vi "Path Edit.vi"() -> ()   [LabVIEW 2016]
uses:
  typedefs/Schedule - enum.ctl
  Global Variables.vi
panel:
  in  "Index":i32=8
  in  "Direction":u16(ring) items=["Forward", "Backward"]
  in  "Enabled":bool=TRUE
  in  "Voltage Schedule":T1
  in  "Apply to All":bool
  in  "Fill Orientation":u16(ring) items=["Horizontal", "Vertical"]
  in  "Smooth Segments":dbl=12.0
  in  "Speed Schedule":T1
  in  "Speed (µm/s)":dbl=8.0
  in  "Voltage (V)":dbl=8.0
  in  "Speed Settings":bool
  in  "Voltage Settings":bool
  in  "Fill Spacing":dbl=0.1
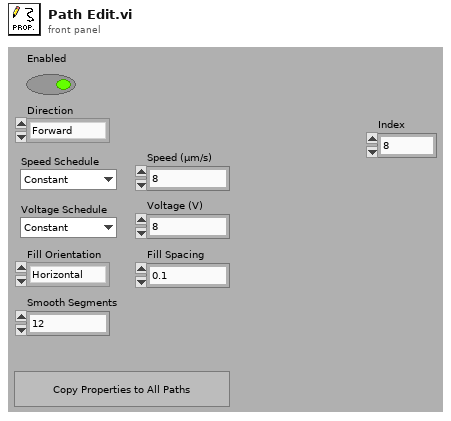
[diagram p1: front panel]
types:
  T1 = typedef "Schedule - enum.ctl" = enum16{"Constant", "Ramp", "Fn. Generator", "Formula"}
  T2 = enum32{"invalid app kind", "Development System", "Run Time System", "Student Edition", "Embedded LabVIEW", "Evaluation", "Custom"}
  T3 = enum32{"Invalid", "Standard", "Closed", "Hidden", "Minimized", "Maximized"}
  T4 = typedef "Path Properties - cluster.ctl" = cluster{"Enabled":bool, "Direction":u16, "Fill Orientation":u16, "Smooth Segments":dbl, "Fill Spacing":dbl, "Speed (um/s)":T5, "Voltage (V)":T5}
  T5 = typedef "Voltage - cluster.ctl" = cluster{"Schedule":T1, "Value":dbl, "Start Value":dbl, "End Value":dbl, "Min Value":dbl, "Max Value":dbl, "Duty Cycle (%)":dbl, "Signal Type":T6, "Cycle Number":dbl, "Phase (degrees)":dbl, "formula":string, "formula length (nm)":dbl, "formula resolution (nm)":dbl}
  T6 = typedef "Signal Type - enum.ctl" = enum16{"Sine Wave", "Triangle Wave", "Square Wave", "Sawtooth Wave"}
  T7 = cluster{"Core":cluster{"Current VI Reference":refnum<vi>, "Close Panel on Exit?":bool}}
  T8 = cluster{"Current VI Reference":refnum<vi>, "Close Panel on Exit?":bool}
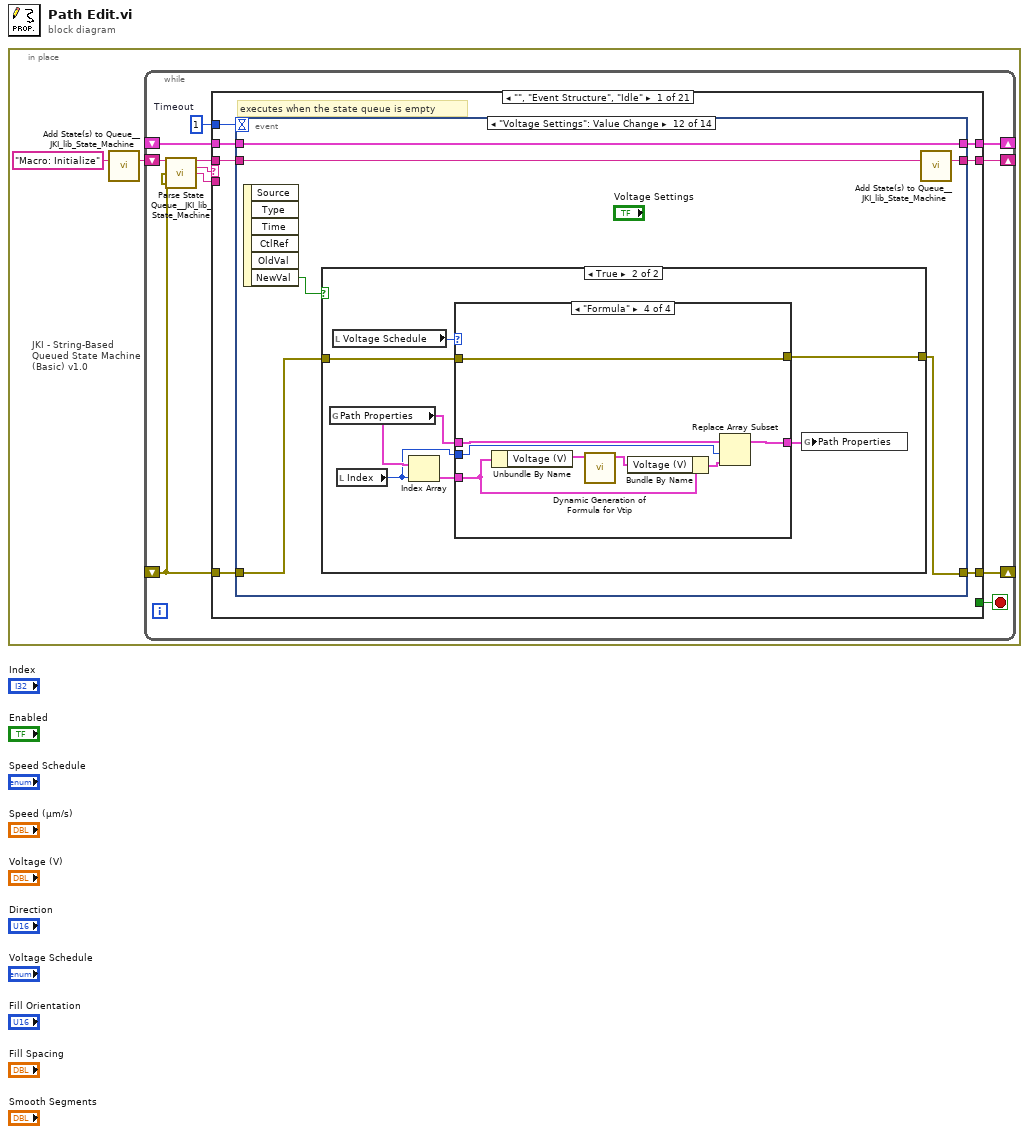
[diagram p0: block diagram]
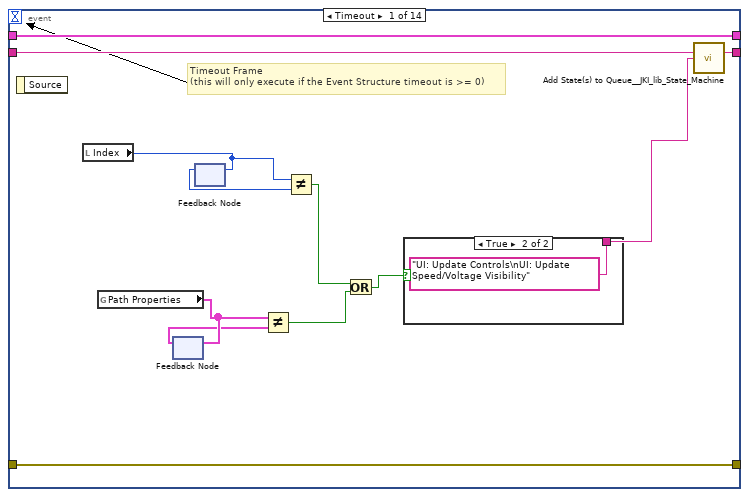
[diagram p2: hidden frame]
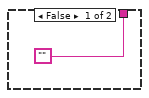
[diagram p3: hidden frame]
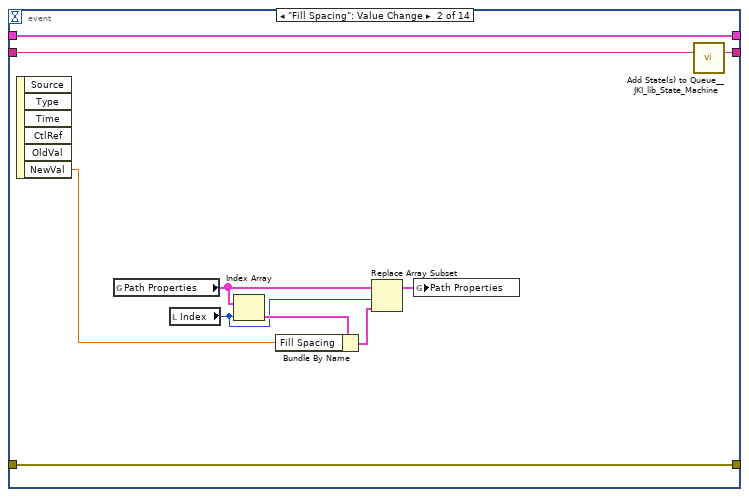
[diagram p4: hidden frame]
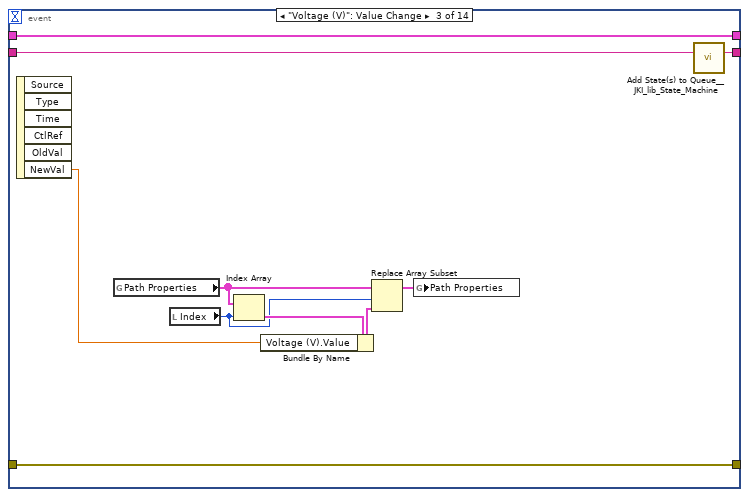
[diagram p5: hidden frame]
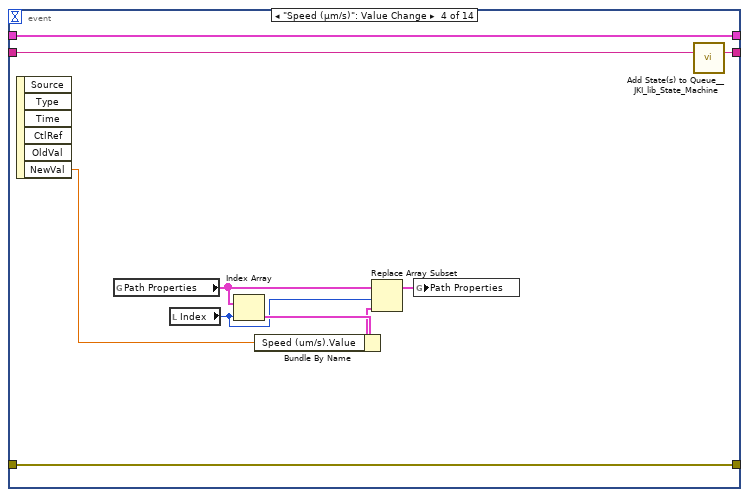
[diagram p6: hidden frame]
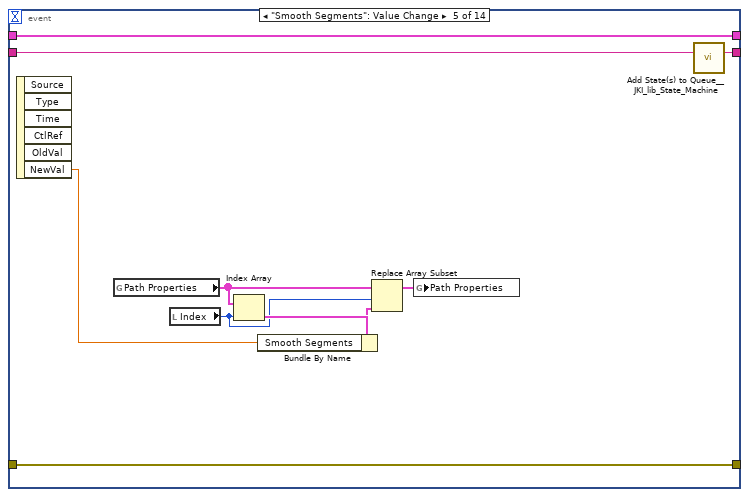
[diagram p7: hidden frame]
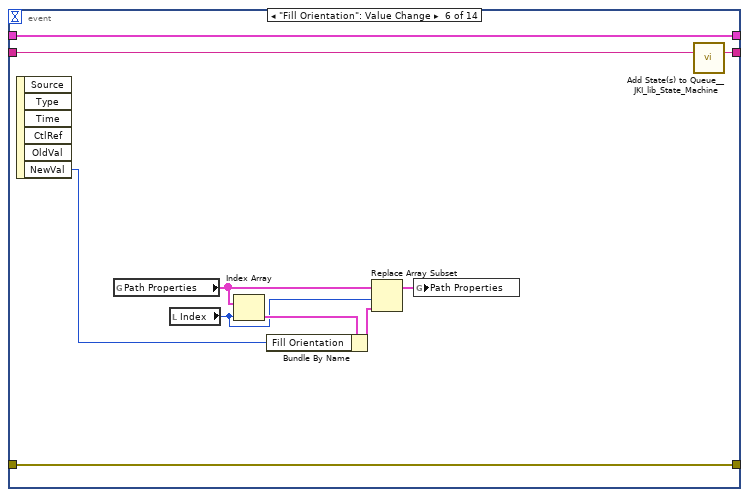
[diagram p8: hidden frame]
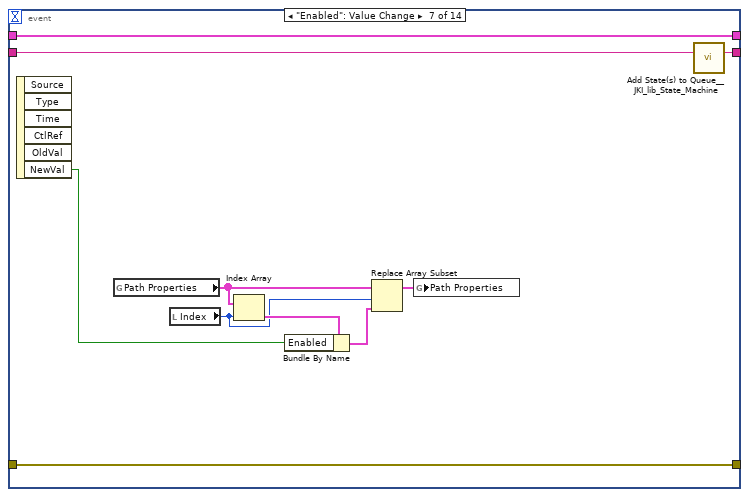
[diagram p9: hidden frame]
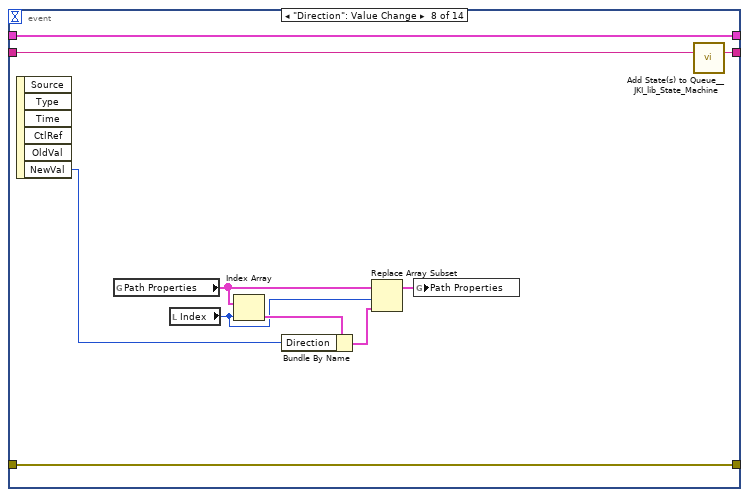
[diagram p10: hidden frame]
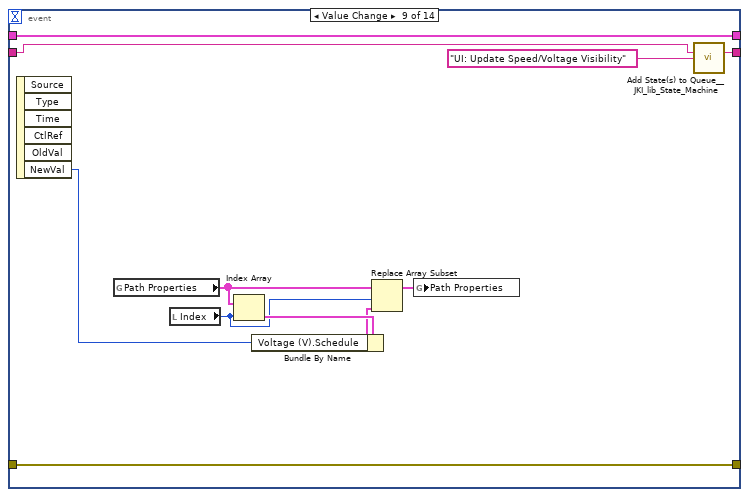
[diagram p11: hidden frame]
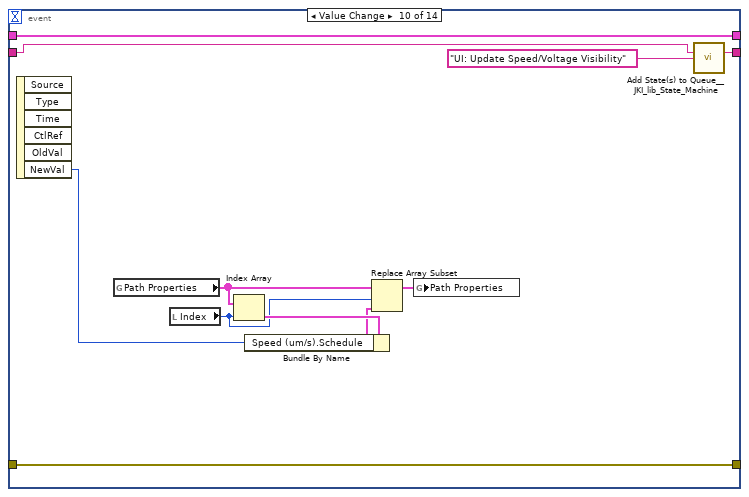
[diagram p12: hidden frame]
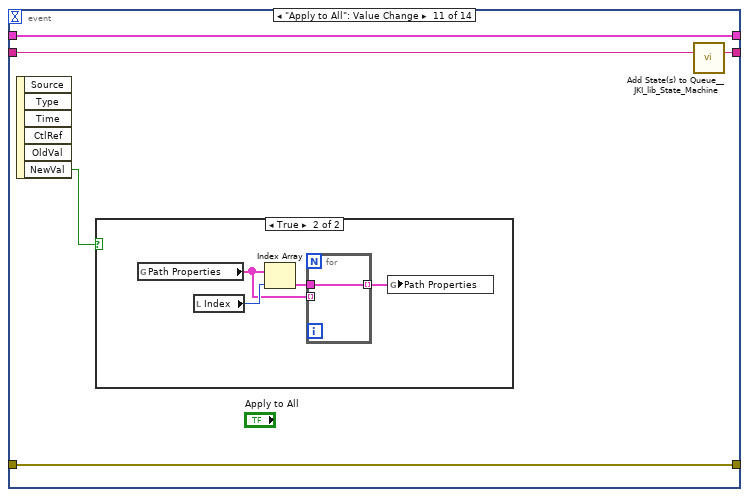
[diagram p13: hidden frame]
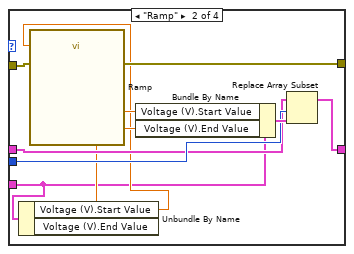
[diagram p17: hidden frame]
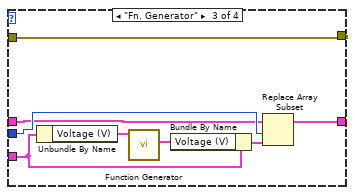
[diagram p18: hidden frame]
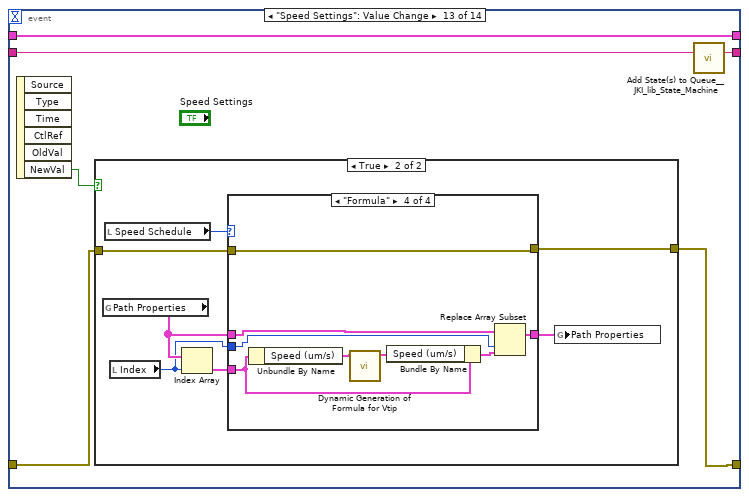
[diagram p19: hidden frame]
diagram:
  n1 = in-place {
    n2 = call <vilib>:"Add State(s) to Queue__JKI_lib_State_Machine.vi"("State(s) in (\"\")"="Macro: Initialize") -> ("States Out"=w2:string)  [unwired: 14 in]
    n3 = while "JKI - String-Based Queued State Machine (Basic) v1.0" {
      shift-right: [w6] -> _
      shift-left: _ -> [w5]
      shift-right: [w9] -> _
      shift-left: _ -> [w3]
      shift-right: [w8] -> _
      shift-left: w2 -> [w10]
      stop <- w7 stop-if-true
      w4 = 1  # Timeout
      n4 = call <vilib>:"Parse State Queue__JKI_lib_State_Machine.vi"("State Queue"=w10, "Error In (no error)"=w3) -> ("Remaining States"=w12:string, "Current State"=w13:string, "Arguments"=w11:string)  [unwired: 11 in]
      n5 = case shown="\"\", \"Event Structure\", \"Idle\"" w13 {
        selector: w13 -> [_ _ w232 _ _ _ _ _ _ _ _ _ _ _ _ _ _ _ _ _ _]
        tunnel: w12 -> [w20 w231 w236 w254 w260 w265 w269 w274 w280 w284 w288 w304 w310 w328 w339 w365 w370 w380 w384 w388 w392]
        tunnel: w11 -> [_ _ _ _ _ _ _ _ _ _ _ _ w305 _ w333 _ _ _ _ _ _]
        tunnel: w5 -> [w18 w228 w234 w250 w257 w263 w266 _ w278 w281 w286 w302 w308 w326 w335 w362 w367 w377 w381 w385 w389]
        tunnel: [w17 w229 w238 w251 errorcluster {"status"=FALSE, "code"=0, "source"=""} ("error out") w262 w267 w270 w276 w282 w285 w301 w306 w315 w336 w363 w368 w378 w382 w386 w390] -> w9
        tunnel: w3 -> [w16 w229 w237 w251 w256 w262 w267 w270 w275 w282 w285 w301 w307 w325 w337 w363 w368 w378 w382 w386 w390]
        tunnel: [w19 w230 w235 w253 w259 w264 w268 w273 w279 w283 w287 w303 w309 w327 w338 w364 w369 w379 w383 w387 w391] -> w8
        tunnel: [_ _ _ _ _ TRUE _ _ _ _ _ _ _ _ _ _ _ _ _ _ _] -> w7
        tunnel: [w15 w228 w234 w252 w257 w263 w266 w272 w278 w281 w286 w302 w308 w326 w335 w362 w367 w377 w381 w385 w389] -> w6
        tunnel: w4 -> [w14 _ _ _ _ _ _ _ _ _ _ _ _ _ _ _ _ _ _ _ _]
        frame "", "Event Structure", "Idle" {
          # "executes when the state queue is empty"
          n6 = event shown="[11] \"Voltage Settings\": Value Change" {
            selector: _ -> [_ _ _ _ _ _ _ _ _ _ _ _ _ _]
            dyn-events: _ -> [_ _ _ _ _ _ _ _ _ _ _ _ _ _]
            timeout: w14 -> [_ _ _ _ _ _ _ _ _ _ _ _ _ _]
            tunnel: w20 -> [w32 w44 w54 w64 w74 w84 w94 w104 w115 w126 w131 w142 w185 w227]
            tunnel: [w31 w43 w53 w63 w73 w83 w93 w103 w114 w125 w130 w141 w184 w226] -> w19
            tunnel: w18 -> [w29 w42 w52 w62 w72 w82 w92 w102 w113 w124 w129 w140 w183 w224]
            tunnel: [w30 w36 w46 w56 w66 w76 w86 w96 w107 w118 w128 w138 w181 w225] -> w17
            tunnel: w16 -> [w30 w36 w46 w56 w66 w76 w86 w96 w107 w118 w128 w139 w182 w225]
            tunnel: [w29 w42 w52 w62 w72 w82 w92 w102 w113 w124 w129 w140 w183 w224] -> w15
            event Timeout {
              # "Timeout Frame\n(this will only execute if the Event Structure timeout is >= 0)"
              n7 = event-data() -> ()  [unwired: 1 in, 1 out]
              n8 = local read "Index"() -> (w27:i32)
              n9 = global read "Global Variables.vi" "Path Properties"() -> (w26:T4[])
              n10 = feedback #1() -> (w25:T4[])  [unwired: 1 in]
              n11 = feedback-in #1(w26) -> ()
              n12 = feedback #2() -> (w28:i32)  [unwired: 1 in]
              n13 = feedback-in #2(w27) -> ()
              n14 = Not Equal?(x=w26, y=w25) -> (x != y?=w23:bool)
              n15 = Not Equal?(x=w27, y=w28) -> (x != y?=w24:bool)
              n16 = Or(x=w24, y=w23) -> (x .or. y?=w22:bool)
              n17 = case shown="True" w22 {
                tunnel: ["" "UI: Update Controls\nUI: Update Speed/Voltage Visibility"] -> w21
                frame False {
                }
                frame True {
                }
              }
              n18 = call <vilib>:"Add State(s) to Queue__JKI_lib_State_Machine.vi"("State(s) in (\"\")"=w32, "State(s) at Back (\"\")"=w21) -> ("States Out"=w31:string)  [unwired: 13 in]
            }
            event "Fill Spacing": Value Change {
              n19 = event-data() -> ("NewVal"=w40:dbl)  [unwired: 1 in, 5 out]
              n20 = global read "Global Variables.vi" "Path Properties"() -> (w38:T4[])
              n21 = local read "Index"() -> (w35:i32)
              n22 = Index Array(array=w38, index=w35) -> (element=w41:T4)
              n23 = Bundle By Name(cluster=w41, "Fill Spacing"=w40) -> (w39:T4)
              n24 = Replace Array Subset(array=w38, new element=w39, index=w35) -> (w37:T4[])
              n25 = global write "Global Variables.vi" "Path Properties"(w37) -> ()
              n26 = call <vilib>:"Add State(s) to Queue__JKI_lib_State_Machine.vi"("State(s) in (\"\")"=w44) -> ("States Out"=w43:string)  [unwired: 14 in]
            }
            event "Voltage (V)": Value Change {
              n27 = event-data() -> ("NewVal"=w50:dbl)  [unwired: 1 in, 5 out]
              n28 = global read "Global Variables.vi" "Path Properties"() -> (w48:T4[])
              n29 = local read "Index"() -> (w45:i32)
              n30 = Index Array(array=w48, index=w45) -> (element=w51:T4)
              n31 = Bundle By Name(cluster=w51, "Voltage (V).Value"=w50) -> (w49:T4)
              n32 = Replace Array Subset(array=w48, new element=w49, index=w45) -> (w47:T4[])
              n33 = global write "Global Variables.vi" "Path Properties"(w47) -> ()
              n34 = call <vilib>:"Add State(s) to Queue__JKI_lib_State_Machine.vi"("State(s) in (\"\")"=w54) -> ("States Out"=w53:string)  [unwired: 14 in]
            }
            event "Speed (µm/s)": Value Change {
              n35 = event-data() -> ("NewVal"=w60:dbl)  [unwired: 1 in, 5 out]
              n36 = global read "Global Variables.vi" "Path Properties"() -> (w58:T4[])
              n37 = local read "Index"() -> (w55:i32)
              n38 = Index Array(array=w58, index=w55) -> (element=w61:T4)
              n39 = Bundle By Name(cluster=w61, "Speed (um/s).Value"=w60) -> (w59:T4)
              n40 = Replace Array Subset(array=w58, new element=w59, index=w55) -> (w57:T4[])
              n41 = global write "Global Variables.vi" "Path Properties"(w57) -> ()
              n42 = call <vilib>:"Add State(s) to Queue__JKI_lib_State_Machine.vi"("State(s) in (\"\")"=w64) -> ("States Out"=w63:string)  [unwired: 14 in]
            }
            event "Smooth Segments": Value Change {
              n43 = event-data() -> ("NewVal"=w70:dbl)  [unwired: 1 in, 5 out]
              n44 = global read "Global Variables.vi" "Path Properties"() -> (w68:T4[])
              n45 = local read "Index"() -> (w65:i32)
              n46 = Index Array(array=w68, index=w65) -> (element=w71:T4)
              n47 = Bundle By Name(cluster=w71, "Smooth Segments"=w70) -> (w69:T4)
              n48 = Replace Array Subset(array=w68, new element=w69, index=w65) -> (w67:T4[])
              n49 = global write "Global Variables.vi" "Path Properties"(w67) -> ()
              n50 = call <vilib>:"Add State(s) to Queue__JKI_lib_State_Machine.vi"("State(s) in (\"\")"=w74) -> ("States Out"=w73:string)  [unwired: 14 in]
            }
            event "Fill Orientation": Value Change {
              n51 = event-data() -> ("NewVal"=w80:u16)  [unwired: 1 in, 5 out]
              n52 = global read "Global Variables.vi" "Path Properties"() -> (w78:T4[])
              n53 = local read "Index"() -> (w75:i32)
              n54 = Index Array(array=w78, index=w75) -> (element=w81:T4)
              n55 = Bundle By Name(cluster=w81, "Fill Orientation"=w80) -> (w79:T4)
              n56 = Replace Array Subset(array=w78, new element=w79, index=w75) -> (w77:T4[])
              n57 = global write "Global Variables.vi" "Path Properties"(w77) -> ()
              n58 = call <vilib>:"Add State(s) to Queue__JKI_lib_State_Machine.vi"("State(s) in (\"\")"=w84) -> ("States Out"=w83:string)  [unwired: 14 in]
            }
            event "Enabled": Value Change {
              n59 = event-data() -> ("NewVal"=w90:bool)  [unwired: 1 in, 5 out]
              n60 = global read "Global Variables.vi" "Path Properties"() -> (w88:T4[])
              n61 = local read "Index"() -> (w85:i32)
              n62 = Index Array(array=w88, index=w85) -> (element=w91:T4)
              n63 = Bundle By Name(cluster=w91, "Enabled"=w90) -> (w89:T4)
              n64 = Replace Array Subset(array=w88, new element=w89, index=w85) -> (w87:T4[])
              n65 = global write "Global Variables.vi" "Path Properties"(w87) -> ()
              n66 = call <vilib>:"Add State(s) to Queue__JKI_lib_State_Machine.vi"("State(s) in (\"\")"=w94) -> ("States Out"=w93:string)  [unwired: 14 in]
            }
            event "Direction": Value Change {
              n67 = event-data() -> ("NewVal"=w100:u16)  [unwired: 1 in, 5 out]
              n68 = global read "Global Variables.vi" "Path Properties"() -> (w98:T4[])
              n69 = local read "Index"() -> (w95:i32)
              n70 = Index Array(array=w98, index=w95) -> (element=w101:T4)
              n71 = Bundle By Name(cluster=w101, "Direction"=w100) -> (w99:T4)
              n72 = Replace Array Subset(array=w98, new element=w99, index=w95) -> (w97:T4[])
              n73 = global write "Global Variables.vi" "Path Properties"(w97) -> ()
              n74 = call <vilib>:"Add State(s) to Queue__JKI_lib_State_Machine.vi"("State(s) in (\"\")"=w104) -> ("States Out"=w103:string)  [unwired: 14 in]
            }
            event Value Change {
              n75 = event-data() -> ("NewVal"=w111:T1)  [unwired: 1 in, 5 out]
              n76 = global read "Global Variables.vi" "Path Properties"() -> (w109:T4[])
              n77 = local read "Index"() -> (w105:i32)
              n78 = Index Array(array=w109, index=w105) -> (element=w112:T4)
              n79 = Bundle By Name(cluster=w112, "Voltage (V).Schedule"=w111) -> (w110:T4)
              n80 = Replace Array Subset(array=w109, new element=w110, index=w105) -> (w108:T4[])
              n81 = global write "Global Variables.vi" "Path Properties"(w108) -> ()
              n82 = call <vilib>:"Add State(s) to Queue__JKI_lib_State_Machine.vi"("State(s) in (\"\")"=w115, "State(s) at Back (\"\")"="UI: Update Speed/Voltage Visibility" ("State(s) at Back (\"\")")) -> ("States Out"=w114:string)  [unwired: 13 in]
            }
            event Value Change {
              n83 = event-data() -> ("NewVal"=w122:T1)  [unwired: 1 in, 5 out]
              n84 = global read "Global Variables.vi" "Path Properties"() -> (w120:T4[])
              n85 = local read "Index"() -> (w116:i32)
              n86 = Index Array(array=w120, index=w116) -> (element=w123:T4)
              n87 = Bundle By Name(cluster=w123, "Speed (um/s).Schedule"=w122) -> (w121:T4)
              n88 = Replace Array Subset(array=w120, new element=w121, index=w116) -> (w119:T4[])
              n89 = global write "Global Variables.vi" "Path Properties"(w119) -> ()
              n90 = call <vilib>:"Add State(s) to Queue__JKI_lib_State_Machine.vi"("State(s) in (\"\")"=w126, "State(s) at Back (\"\")"="UI: Update Speed/Voltage Visibility" ("State(s) at Back (\"\")")) -> ("States Out"=w125:string)  [unwired: 13 in]
            }
            event "Apply to All": Value Change {
              n91 = event-data() -> ("NewVal"=w127:bool)  [unwired: 1 in, 5 out]
              n92 = case shown="True" w127 {
                frame False {
                }
                frame True {
                  n93 = global read "Global Variables.vi" "Path Properties"() -> (w132:T4[])
                  n94 = local read "Index"() -> (w135:i32)
                  n95 = Index Array(array=w132, index=w135) -> (element=w134:T4)
                  n96 = for {
                    tunnel: w134 -> [w136]
                    tunnel: [w136] -> w133 mode=indexing
                    tunnel: w132 -> [_] mode=indexing
                  }
                  n97 = global write "Global Variables.vi" "Path Properties"(w133) -> ()
                }
              }
              n98 = call <vilib>:"Add State(s) to Queue__JKI_lib_State_Machine.vi"("State(s) in (\"\")"=w131) -> ("States Out"=w130:string)  [unwired: 14 in]
            }
            event "Voltage Settings": Value Change {
              n99 = event-data() -> ("NewVal"=w137:bool)  [unwired: 1 in, 5 out]
              n100 = case shown="True" w137 {
                tunnel: w139 -> [w143 w149]
                tunnel: [w143 w148] -> w138
                frame False {
                }
                frame True {
                  n101 = global read "Global Variables.vi" "Path Properties"() -> (w145:T4[])
                  n102 = local read "Voltage Schedule"() -> (w150:T1)
                  n103 = local read "Index"() -> (w144:i32)
                  n104 = Index Array(array=w145, index=w144) -> (element=w146:T4)
                  n105 = case shown="\"Formula\"" w150 {
                    tunnel: w149 -> [w152 w163 w167 w179]
                    tunnel: [w152 w156 w167 w179] -> w148
                    tunnel: [w151 w157 w168 w172] -> w147
                    tunnel: w146 -> [_ w153 w166 w177]
                    tunnel: w145 -> [w151 w158 w169 w176]
                    tunnel: w144 -> [_ w159 w170 w175]
                    frame "Constant", Default {
                    }
                    frame "Ramp" {
                      n106 = Unbundle By Name(w153) -> ("Voltage (V).Start Value"=w155:dbl, "Voltage (V).End Value"=w154:dbl)
                      n107 = call "Ramp.vi"("Start Value"=w155, "End Value"=w154, "error in (no error)"=w163) -> ("End Value"=w161:dbl, "Start Value"=w162:dbl, "error out"=w156:errorcluster)  [unwired: 13 in, 1 out]
                      n108 = Bundle By Name(cluster=w153, "Voltage (V).Start Value"=w162, "Voltage (V).End Value"=w161) -> (w160:T4)
                      n109 = Replace Array Subset(array=w158, new element=w160, index=w159) -> (w157:T4[])
                    }
                    frame "Fn. Generator" {
                      n110 = Unbundle By Name(w166) -> ("Voltage (V)"=w164:T5)
                      n111 = call "Function Generator.vi"("Properties in"=w164) -> ("Properties out"=w165:T5)  [unwired: 9 in, 1 out]
                      n112 = Bundle By Name(cluster=w166, "Voltage (V)"=w165) -> (w171:T4)
                      n113 = Replace Array Subset(array=w169, new element=w171, index=w170) -> (w168:T4[])
                    }
                    frame "Formula" {
                      n114 = Unbundle By Name(w177) -> ("Voltage (V)"=w174:T5)
                      n115 = call "Dynamic Generation of Formula for Vtip.vi"("Voltage (V)"=w174) -> ("Voltage (V) 2"=w173:T5)  [unwired: 10 in]
                      n116 = Bundle By Name(cluster=w177, "Voltage (V)"=w173) -> (w178:T4)
                      n117 = Replace Array Subset(array=w176, new element=w178, index=w175) -> (w172:T4[])
                    }
                  }
                  n118 = global write "Global Variables.vi" "Path Properties"(w147) -> ()
                }
              }
              n119 = call <vilib>:"Add State(s) to Queue__JKI_lib_State_Machine.vi"("State(s) in (\"\")"=w142) -> ("States Out"=w141:string)  [unwired: 14 in]
            }
            event "Speed Settings": Value Change {
              n120 = event-data() -> ("NewVal"=w180:bool)  [unwired: 1 in, 5 out]
              n121 = case shown="True" w180 {
                tunnel: w182 -> [w186 w192]
                tunnel: [w186 w191] -> w181
                frame False {
                }
                frame True {
                  n122 = global read "Global Variables.vi" "Path Properties"() -> (w188:T4[])
                  n123 = local read "Speed Schedule"() -> (w193:T1)
                  n124 = local read "Index"() -> (w187:i32)
                  n125 = Index Array(array=w188, index=w187) -> (element=w189:T4)
                  n126 = case shown="\"Formula\"" w193 {
                    tunnel: w192 -> [w195 _ w209 w221]
                    tunnel: [w195 w201 w209 w221] -> w191
                    tunnel: [w194 w200 w210 w214] -> w190
                    tunnel: w189 -> [_ w196 w208 w218]
                    tunnel: w188 -> [w194 w198 w211 w219]
                    tunnel: w187 -> [_ w199 w212 w217]
                    frame "Constant", Default {
                    }
                    frame "Ramp" {
                      n127 = Unbundle By Name(w196) -> ("Speed (um/s).Start Value"=w202:dbl, "Speed (um/s).End Value"=w197:dbl)
                      n128 = call "Ramp.vi"("Start Value"=w202, "End Value"=w197) -> ("End Value"=w204:dbl, "Start Value"=w205:dbl, "error out"=w201:errorcluster)  [unwired: 14 in, 1 out]
                      n129 = Bundle By Name(cluster=w196, "Speed (um/s).Start Value"=w205, "Speed (um/s).End Value"=w204) -> (w203:T4)
                      n130 = Replace Array Subset(array=w198, new element=w203, index=w199) -> (w200:T4[])
                    }
                    frame "Fn. Generator" {
                      n131 = Unbundle By Name(w208) -> ("Speed (um/s)"=w206:T5)
                      n132 = call "Function Generator.vi"("Properties in"=w206) -> ("Properties out"=w207:T5)  [unwired: 9 in, 1 out]
                      n133 = Bundle By Name(cluster=w208, "Speed (um/s)"=w207) -> (w213:T4)
                      n134 = Replace Array Subset(array=w211, new element=w213, index=w212) -> (w210:T4[])
                    }
                    frame "Formula" {
                      n135 = Unbundle By Name(w218) -> ("Speed (um/s)"=w215:T5)
                      n136 = call "Dynamic Generation of Formula for Vtip.vi"("Voltage (V)"=w215) -> ("Voltage (V) 2"=w216:T5)  [unwired: 10 in]
                      n137 = Bundle By Name(cluster=w218, "Speed (um/s)"=w216) -> (w220:T4)
                      n138 = Replace Array Subset(array=w219, new element=w220, index=w217) -> (w214:T4[])
                    }
                  }
                  n139 = global write "Global Variables.vi" "Path Properties"(w190) -> ()
                }
              }
              n140 = call <vilib>:"Add State(s) to Queue__JKI_lib_State_Machine.vi"("State(s) in (\"\")"=w185) -> ("States Out"=w184:string)  [unwired: 14 in]
            }
            event Panel Close? {
              # "Discard the event because we'll close the front panel ourselves in Macro: Exit"
              # "Close Panel button (pressed) Event\n(this executes Macro: Exit to terminate the VI)"
              n141 = event-data() -> ()  [unwired: 1 in, 1 out]
              n142 = event-data("Discard?"=TRUE) -> ()  [unwired: 1 in, 1 out]
              n143 = call <vilib>:"Add State(s) to Queue__JKI_lib_State_Machine.vi"("State(s) in Front (\"\")"="Macro: Exit", "State(s) in (\"\")"=w227) -> ("States Out"=w226:string)  [unwired: 13 in]
            }
          }
        }
        frame "---------- Core ----------" {
          # "Do not put any code in this frame.\n(it is a separator no-op)"
          n144 = call <vilib>:"Add State(s) to Queue__JKI_lib_State_Machine.vi"("State(s) in (\"\")"=w231) -> ("States Out"=w230:string)  [unwired: 14 in]
        }
        frame Default {
          w241 = 42 items=["No error", "Argument error", "Memory is full", "Out of zone", "End of file", "File already open", "Generic file I/O error", "File not found", "File permission error", "Disk is full", "Duplicate path", "Too many files open", "System feature not enabled", "Resource file not found", "Cannot add resource", "Resource not found", "Image not found", "Image memory error", "Pen does not exist", "Config type invalid", "Config token not found", "Config parse error", "Config memory error", "Bad external code format", "Bad external code offset", "External code not present", "Null window", "Destroy window error", "Null menu", "Print aborted", "Bad print record", "Print driver error", "Windows error during printing", "Memory error during printing", "Print dialog error", "Generic print error", "Invalid device refnum", "Device not found", "Device parameter error", "Device unit error", "Cannot open device", "Device call aborted", "Generic error", "Cancelled by user", "Object ID too low", "Object ID too high", "Object not in heap", "Unknown heap", "Unknown object (invalid DefProc)", "Unknown object (DefProc not in table)", "Message out of range", "Invalid (null) method", "Unknown message", "Manager call not supported", "Bad address", "Network operation in progress", "Network operation timed out", "Connection is busy", "Network attribute not supported", "Network error", "Address in use", "System out of memory", "Connection aborted", "Connection refused", "Not connected", "Already connected", "Connection closed", "Initialization error (interapplication manager)", "Bad occurrence", "Wait on unbound occurrence handler", "Occurrence queue overflow", "Datalog type conflict", "Unused", "Unrecognized type (interapplication manager)", "Memory corrupt", "Failed to make temporary DLL", "Old CIN version", "Drag socket not found", "Failed to load drop-object", "Failed to register OLE object", "Failed to release OLE object", "Format specifier type mismatch", "Unknown format specifier", "Too few format specifiers", "Too many format specifiers", "Scan failed", "Newer CIN version", "Error converting to variant", "Runtime menu error", "Password tampered", "Variant attribute not found", "Incompatible variant data type", "Event data is not available", "Event Store is not present", "Occurrence is not found", "Event Queue is not created", "Event info is not available", "Refnum passed is NULL", "Error retrieving Class GUID", "Error retrieving CoClass GUID", "Error retrieving TypeLib GUID.", "Bad built application magic bytes.", "Specific driver is different from the specific driver associated with the Logical Name.", "There is no session opened to the class driver.", "Max Error", "MAX - Error with config objects", "MAX - Error loading configuration", "MAX - Group not supported"]
          # "Current State"
          # "Do not delete, rename, or modify this frame.\n(this is used to capture unhandled states and typos)"
          # "Handle mistyped state name (developer tool)"
          n145 = Format Into String(format string="Software Exception: Unhandled State \"%s\"." ("message"), error in=w237, w232) -> (resulting string=w240:string, error out=w239:errorcluster)  [unwired: 1 in]
          n146 = call <vilib>:"Error Cluster From Error Code.vi"("show call chain? (False)"=TRUE, "error in (no error)"=w239, "error message (\"\")"=w240, "error code (0)"=w241) -> ("error out"=w238:errorcluster)  [unwired: 5 in]
          n147 = call <vilib>:"Add State(s) to Queue__JKI_lib_State_Machine.vi"("State(s) in (\"\")"=w236) -> ("States Out"=w235:string)  [unwired: 14 in]
        }
        frame "Initialize Core Data" {
          # "exe?"
          # "If panel starts closed or is an EXE, then close it when we exit"
          # "Do not delete, rename, or modify this frame.\n(this is used to determine panel behavior on exit)"
          n148 = control-ref of="Current VI Reference"() -> (w249:refnum<vi>)
          n149 = property class="VI"() -> ("Front Panel.Open"=w248:bool)  [unwired: 2 in, 2 out]
          n150 = property class="App"() -> ("App.Kind"=w247:T2)  [unwired: 2 in, 2 out]
          n151 = Not(x=w248) -> (.not. x?=w245:bool)
          n152 = Equal?(x=w247, y=T2."Run Time System" ("Application:Kind")) -> (x = y?=w244:bool)
          n153 = Or(x=w245, y=w244) -> (x .or. y?=w243:bool)
          n154 = Bundle By Name(cluster=w250, "Core.Current VI Reference"=w249, "Core.Close Panel on Exit?"=w243) -> (w252:T7)
          n155 = call <vilib>:"Add State(s) to Queue__JKI_lib_State_Machine.vi"("State(s) in (\"\")"=w254) -> ("States Out"=w253:string)  [unwired: 14 in]
        }
        frame "Error Handler" {
          # "Unhandled Error -- Display it"
          # "Handle any errors here.\nYou can also output any states to clean-up after errors occur"
          # "Clear error"
          n156 = call <vilib>:"General Error Handler.vi"("error in (no error)"=w256) -> ()  [unwired: 10 in, 5 out]
          n157 = call <vilib>:"Add State(s) to Queue__JKI_lib_State_Machine.vi"("State(s) in Front (\"\")"="/* Post Error States", "State(s) in (\"\")"=w260) -> ("States Out"=w259:string)  [unwired: 13 in]
        }
        frame "Exit" {
          # "Do not put any code in this frame.\n(No errors that occur here will be handled.)"
          n158 = call <vilib>:"Add State(s) to Queue__JKI_lib_State_Machine.vi"("State(s) in (\"\")"=w265) -> ("States Out"=w264:string)  [unwired: 14 in]
        }
        frame "---------- Data ----------" {
          # "Do not put any code in this frame.\n(It is a separator no-op. You can make a copy of this frame to create a new Data frame)"
          n159 = call <vilib>:"Add State(s) to Queue__JKI_lib_State_Machine.vi"("State(s) in (\"\")"=w269) -> ("States Out"=w268:string)  [unwired: 14 in]
        }
        frame "Data: Initialize" {
          w271 = T8 {"Current VI Reference"=refnum, "Close Panel on Exit?"=FALSE}  # Core
          # "Initialize the shift-register data, here.\n(data names are defined by what you wire into the bundle function)"
          n160 = Bundle("Core"=w271) -> (w272:T7)  [unwired: 1 in]
          n161 = call <vilib>:"Add State(s) to Queue__JKI_lib_State_Machine.vi"("State(s) in (\"\")"=w274) -> ("States Out"=w273:string)  [unwired: 14 in]
        }
        frame "Data: Cleanup" {
          # "Cleanup any data and references, here.\n(this is called automatically, by the Macro: Exit)"
          n162 = Unbundle By Name(w278) -> ("Core.Current VI Reference"=w277:refnum<vi>)
          n163 = Close Reference(reference=w277, error in (no error)=w275) -> (error out=w276:errorcluster)
          n164 = call <vilib>:"Add State(s) to Queue__JKI_lib_State_Machine.vi"("State(s) in (\"\")"=w280) -> ("States Out"=w279:string)  [unwired: 14 in]
        }
        frame "---------- UI ----------" {
          # "Do not put any code in this frame.\n(It is a separator no-op. You can make a copy of this frame to create a new UI frame)"
          n165 = call <vilib>:"Add State(s) to Queue__JKI_lib_State_Machine.vi"("State(s) in (\"\")"=w284) -> ("States Out"=w283:string)  [unwired: 14 in]
        }
        frame "UI: Initialize" {
          # "Initialize the User Interface, here.\n(this is called automatically, by the Macro: Init)"
          n166 = call <vilib>:"Add State(s) to Queue__JKI_lib_State_Machine.vi"("State(s) in (\"\")"=w288) -> ("States Out"=w287:string)  [unwired: 14 in]
        }
        frame "UI: Update Controls" {
          n167 = global read "Global Variables.vi" "Path Properties"() -> (w289:T4[])
          n168 = local read "Index"() -> (w293:i32)
          n169 = Index Array(array=w289, index=w293) -> (element=w292:T4)
          n170 = Unbundle By Name(w292) -> ("Enabled"=w294:bool, "Direction"=w295:u16, "Fill Orientation"=w296:u16, "Smooth Segments"=w297:dbl, "Fill Spacing"=w298:dbl, "Speed (um/s).Schedule"=w291:T1, "Speed (um/s).Value"=w299:dbl, "Voltage (V).Schedule"=w290:T1, "Voltage (V).Value"=w300:dbl)
          n171 = local write "Enabled"(w294) -> ()
          n172 = local write "Direction"(w295) -> ()
          n173 = local write "Fill Orientation"(w296) -> ()
          n174 = local write "Smooth Segments"(w297) -> ()
          n175 = local write "Fill Spacing"(w298) -> ()
          n176 = local write "Speed Schedule"(w291) -> ()
          n177 = local write "Speed (µm/s)"(w299) -> ()
          n178 = local write "Voltage Schedule"(w290) -> ()
          n179 = local write "Voltage (V)"(w300) -> ()
          n180 = call <vilib>:"Add State(s) to Queue__JKI_lib_State_Machine.vi"("State(s) in (\"\")"=w304) -> ("States Out"=w303:string)  [unwired: 14 in]
        }
        frame "UI: Cursor Set" {
          # "Argument"
          # "Set and Unset Cursor Busy.\n(Usage: \"UI: Cursor Set >> Busy|Idle\")"
          n181 = case shown="\"Idle\", Default" w305 {
            tunnel: w307 -> [w312 w314]
            tunnel: [w311 w313] -> w306
            frame "Idle", Default {
              n182 = call <vilib>:"Unset Busy.vi"("error in (no error)"=w312) -> ("error out"=w311:errorcluster)  [unwired: 10 in]
            }
            frame "Busy" {
              n183 = call <vilib>:"Set Busy.vi"("error in (no error)"=w314) -> ("error out"=w313:errorcluster)  [unwired: 9 in, 1 out]
            }
          }
          n184 = call <vilib>:"Add State(s) to Queue__JKI_lib_State_Machine.vi"("State(s) in (\"\")"=w310) -> ("States Out"=w309:string)  [unwired: 14 in]
        }
        frame "UI: Update Speed/Voltage Visibility" {
          n185 = local read "Voltage Schedule"() -> (w324:T1)
          n186 = local read "Speed Schedule"() -> (w323:T1)
          n187 = case shown="\"Ramp\", Default" w324 {
            tunnel: [TRUE FALSE] -> w320
            frame "Constant" {
            }
            frame "Ramp", Default {
            }
          }
          n188 = property on="Voltage (V)" class="DigNum (strict)"(error in=w325, "Visible"=w320) -> (error out=w321:errorcluster)  [unwired: 1 in, 1 out]
          n189 = case shown="\"Ramp\", Default" w323 {
            tunnel: [TRUE FALSE] -> w316
            frame "Constant" {
            }
            frame "Ramp", Default {
            }
          }
          n190 = Not(x=w320) -> (.not. x?=w319:bool)
          n191 = property on="Voltage Settings" class="Bool"(error in=w321, "Visible"=w319) -> (error out=w318:errorcluster)  [unwired: 1 in, 1 out]
          n192 = property on="Speed (µm/s)" class="DigNum (strict)"(error in=w318, "Visible"=w316) -> (error out=w317:errorcluster)  [unwired: 1 in, 1 out]
          n193 = Not(x=w316) -> (.not. x?=w322:bool)
          n194 = property on="Speed Settings" class="Bool"(error in=w317, "Visible"=w322) -> (error out=w315:errorcluster)  [unwired: 1 in, 1 out]
          n195 = call <vilib>:"Add State(s) to Queue__JKI_lib_State_Machine.vi"("State(s) in (\"\")"=w328) -> ("States Out"=w327:string)  [unwired: 14 in]
        }
        frame "UI: Front Panel State" {
          # "Argument"
          # "Set Front Panel Open or Closed\n(Usage: \"UI: Front Panel State >> Open|Close\")"
          n196 = Unbundle By Name(w335) -> ("Core.Current VI Reference"=w334:refnum<vi>)
          n197 = case shown="\"Open\", Default" w333 {
            tunnel: w337 -> [w343 w356]
            tunnel: [w345 w357] -> w336
            tunnel: w334 -> [w344 w354]
            frame "Open", Default {
              n198 = property class="VI"(reference=w344, error in=w343) -> (reference out=w341:refnum<vi>, error out=w342:errorcluster, "Front Panel.Open"=w340:bool)
              n199 = case shown="False" w340 {
                tunnel: [w348 w351] -> w345
                tunnel: w342 -> [w347 w351]
                tunnel: w341 -> [w346 _]
                frame False {
                  n200 = invoke class="VI" method="FP.Open"(reference=w346, error in=w347, "Activate"=TRUE, "State"=T3."Standard") -> (error out=w348:errorcluster)  [unwired: 1 in, 4 out]
                }
                frame True {
                }
              }
            }
            frame "Close" {
              n201 = property class="VI"(reference=w354, error in=w356) -> (reference out=w353:refnum<vi>, error out=w355:errorcluster, "Front Panel.Open"=w352:bool)
              n202 = case shown="True" w352 {
                tunnel: [w358 w361] -> w357
                tunnel: w355 -> [w358 w360]
                tunnel: w353 -> [_ w359]
                frame False {
                }
                frame True {
                  n203 = invoke class="VI" method="FP.Close"(reference=w359, error in=w360) -> (error out=w361:errorcluster)  [unwired: 1 in, 2 out]
                }
              }
            }
          }
          n204 = call <vilib>:"Add State(s) to Queue__JKI_lib_State_Machine.vi"("State(s) in (\"\")"=w339) -> ("States Out"=w338:string)  [unwired: 14 in]
        }
        frame "---------- Macro ----------" {
          # "Do not put any code in this frame.\n(It is a separator no-op. You can make a copy of this frame to create a new Macro frame)"
          n205 = call <vilib>:"Add State(s) to Queue__JKI_lib_State_Machine.vi"("State(s) in (\"\")"=w365) -> ("States Out"=w364:string)  [unwired: 14 in]
        }
        frame "Macro: Initialize" {
          w366 = "Data: Initialize\nInitialize Core Data\nUI: Initialize\nUI: Update Controls\nUI: Update Speed/Voltage Visibility\nUI: Front Panel State >> Close"  # Data: Initialize Initialize Core Data UI: Initialize UI: Update Controls UI: Update Speed/Voltage Visibility UI: Front Panel State >> Close
          # "Initialization Macro\n(This is called once, when the VI starts)"
          n206 = call <vilib>:"Add State(s) to Queue__JKI_lib_State_Machine.vi"("State(s) in Front (\"\")"=w366, "State(s) in (\"\")"=w370) -> ("States Out"=w369:string)  [unwired: 13 in]
        }
        frame "Macro: Exit" {
          # "Exit Macro\n(This is called once, when the VI exits)"
          n207 = Unbundle By Name(w377) -> ("Core.Close Panel on Exit?"=w376:bool)
          n208 = Select(t="UI: Front Panel State >> Close", s=w376, f="") -> (s? t:f=w373:string)
          n209 = call <vilib>:"Add State(s) to Queue__JKI_lib_State_Machine.vi"("State(s) in (\"\")"=w373, "State(s) at Back (\"\")"="Data: Cleanup\nExit") -> ("States Out"=w371:string)  [unwired: 13 in]
          n210 = call <vilib>:"Add State(s) to Queue__JKI_lib_State_Machine.vi"("State(s) in Front (\"\")"=w371, "State(s) in (\"\")"=w380) -> ("States Out"=w379:string)  [unwired: 13 in]
        }
        frame "---------- New Category ----------" {
          # "Template Separator\n(You can make a copy of, or modify, this frame)"
          n211 = call <vilib>:"Add State(s) to Queue__JKI_lib_State_Machine.vi"("State(s) in (\"\")"=w384) -> ("States Out"=w383:string)  [unwired: 14 in]
        }
        frame "New Category: 1" {
          # "Your code here.\n(You can make a copy of, or modify, this frame)"
          n212 = call <vilib>:"Add State(s) to Queue__JKI_lib_State_Machine.vi"("State(s) in (\"\")"=w388) -> ("States Out"=w387:string)  [unwired: 14 in]
        }
        frame "New Category: 2" {
          # "Your code here.\n(You can make a copy of, or modify, this frame)"
          n213 = call <vilib>:"Add State(s) to Queue__JKI_lib_State_Machine.vi"("State(s) in (\"\")"=w392) -> ("States Out"=w391:string)  [unwired: 14 in]
        }
      }
    }
  }
